vi "ALPErrToHumanReadable.vi"(10 "Error In":string[](array[string]), 11 "Error Codes":dbl[](array[numeric])) -> (3 "Error Out":string[](array[string]))   [LabVIEW 2013, in "alpD41.lvlib"]
uses:
  alpD41.lvlib
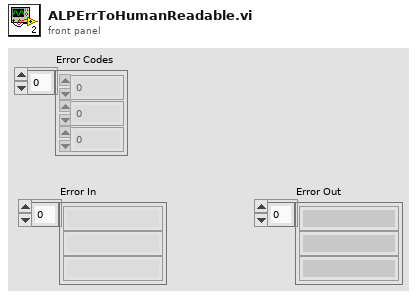
[diagram p1: front panel]
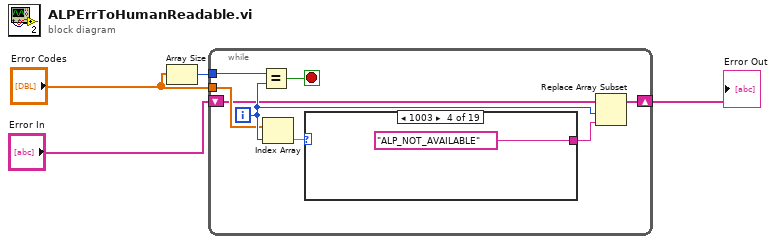
[diagram p0: block diagram]
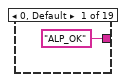
[diagram p2: hidden frame]
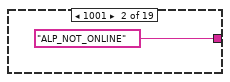
[diagram p3: hidden frame]
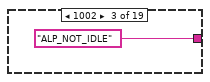
[diagram p4: hidden frame]
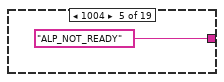
[diagram p5: hidden frame]
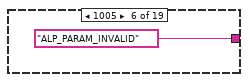
[diagram p6: hidden frame]
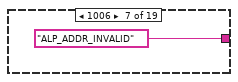
[diagram p7: hidden frame]
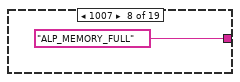
[diagram p8: hidden frame]
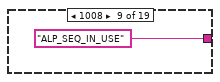
[diagram p9: hidden frame]
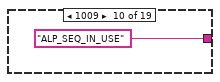
[diagram p10: hidden frame]
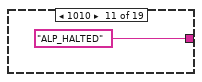
[diagram p11: hidden frame]
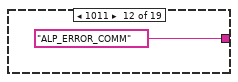
[diagram p12: hidden frame]
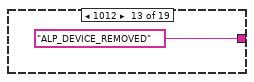
[diagram p13: hidden frame]
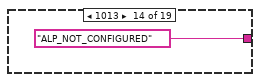
[diagram p14: hidden frame]
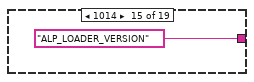
[diagram p15: hidden frame]
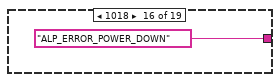
[diagram p16: hidden frame]
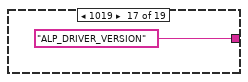
[diagram p17: hidden frame]
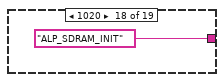
[diagram p18: hidden frame]
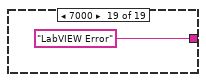
[diagram p19: hidden frame]
diagram:
  n1 = Array Size(array="Error Codes") -> (size(s)=w4:i32)
  n2 = while {
    tunnel: w4 -> [w11]
    tunnel: "Error Codes" -> [w7]
    shift-right: [w5] -> w1
    shift-left: "Error In" -> [w6]
    i -> [w8]
    stop <- w12 stop-if-true
    n3 = Equal?(x=w11, y=w8) -> (x = y?=w12:bool)
    n4 = Index Array(array=w7, index=w8) -> (element=w10:dbl)
    n5 = case shown="1003" w10 {
      tunnel: ["ALP_OK" "ALP_NOT_ONLINE" "ALP_NOT_IDLE" "ALP_NOT_AVAILABLE" "ALP_NOT_READY" "ALP_PARAM_INVALID" "ALP_ADDR_INVALID" "ALP_MEMORY_FULL" "ALP_SEQ_IN_USE" "ALP_SEQ_IN_USE" "ALP_HALTED" "ALP_ERROR_COMM" "ALP_DEVICE_REMOVED" "ALP_NOT_CONFIGURED" "ALP_LOADER_VERSION" "ALP_ERROR_POWER_DOWN" "ALP_DRIVER_VERSION" "ALP_SDRAM_INIT" "LabVIEW Error"] -> w9
      frame 0, Default {
      }
      frame 1001 {
      }
      frame 1002 {
      }
      frame 1003 {
      }
      frame 1004 {
      }
      frame 1005 {
      }
      frame 1006 {
      }
      frame 1007 {
      }
      frame 1008 {
      }
      frame 1009 {
      }
      frame 1010 {
      }
      frame 1011 {
      }
      frame 1012 {
      }
      frame 1013 {
      }
      frame 1014 {
      }
      frame 1018 {
      }
      frame 1019 {
      }
      frame 1020 {
      }
      frame 7000 {
      }
    }
    n6 = Replace Array Subset(array=w6, new element=w9, index=w8) -> (w5:string[])
  }
  "Error Out" <- w1
